vi "5.7.4-UDP-OCU_to_Forbrain-Client.vi"() -> ()   [LabVIEW 2010]
doc: "This VI implements a client for the Named Service UDP Server.vi.\nIt connects to a service by specifying the server address and the name of the service. After sending a 'Hello' string to the server, the client receives the string sent by the server, displays the string and closes the connection.\n\n<b>Note:</b> This VI is built to work with the Named Service UDP Server.vi in UDP.llb."
uses:
  6-OCU Neurons/AutoModeControls.ctl
  5.0-Global.vi
panel:
  out "AutoModeDatums":T1
  out "String":string
  out "error out":errorcluster
  in  "error in":errorcluster
  # "Instructions:\n1. Open Named Service UDP Server.vi located in the same library.\n2. Follow the instructions on it's front panel.\n\nNote: This VI is built to work with the Named Service UDP Server.vi in UDP.llb."
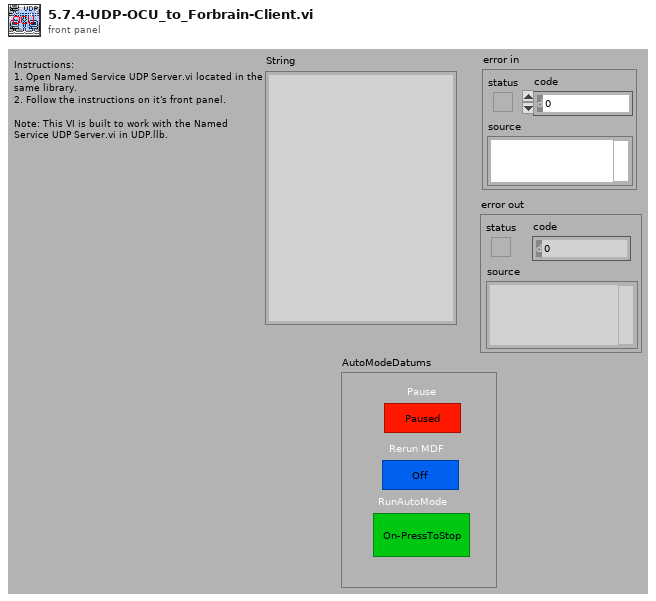
[diagram p1: front panel]
types:
  T1 = typedef "AutoModeControls.ctl" = cluster{"RunAutoMode":bool, "Rerun MDF":bool, "Pause":bool}
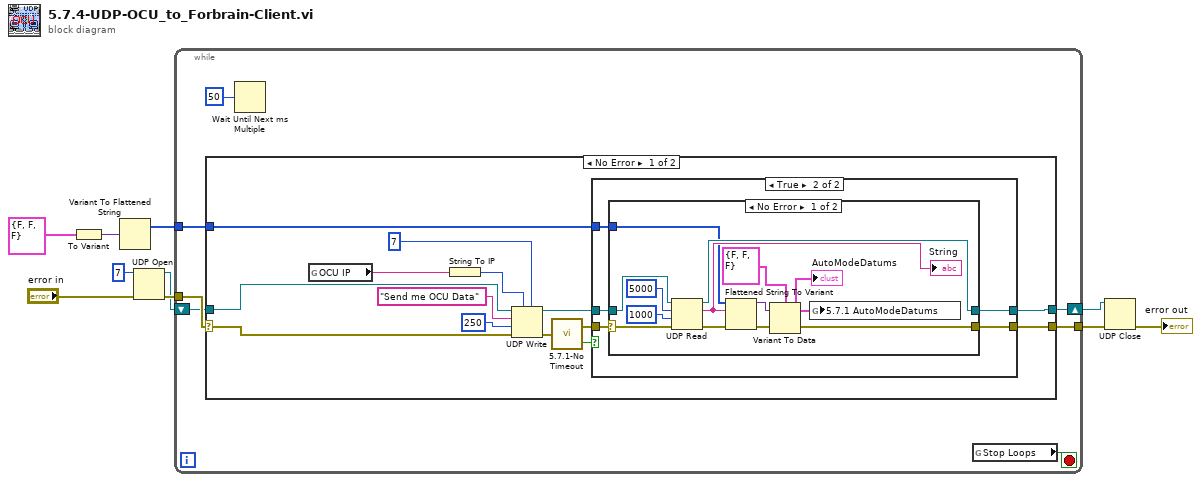
[diagram p0: block diagram]
diagram:
  n1 = To Variant(anything=T1 {"RunAutoMode"=FALSE, "Rerun MDF"=FALSE, "Pause"=FALSE} ("AutoModeDatums")) -> (Variant=w4:variant)
  n2 = Variant To Flattened String(Variant=w4) -> (1:w3:i16[])  [unwired: 1 out]
  n3 = UDP Open(8:"error in", 11:u16 7 ("port")) -> (port=w8:refnum<k16>, 0:w9:errorcluster)  [unwired: 3 in, 1 out]
  n4 = while {
    tunnel: [w17] -> w6
    tunnel: w9 -> [w16]
    shift-right: [w14] -> w7
    shift-left: w8 -> [w15]
    tunnel: w3 -> [w12]
    stop <- w11 stop-if-true
    n5 = case shown="No Error" w16 {
      selector: w16 -> [w31 w55]
      tunnel: [w26 w55] -> w17
      tunnel: w15 -> [w30 w54]
      tunnel: [w25 w54] -> w14
      tunnel: w12 -> [w20 _]
      frame No Error {
        n6 = global read "5.0-Global.vi" "OCU IP"() -> (w19:string)
        n7 = String To IP(1:w19) -> (0:w29:u32)
        n8 = UDP Write(address=w29, port or service name=u16 7, connection ID=w30, data in="Send me OCU Data", 8:w31, 9:250 ("timeout ms (25000)")) -> (error out=w24:errorcluster, 3:w27:refnum<k16>)
        n9 = call "5.7.1-No Timeout.vi"("error in (no error)"=w24) -> ("No Timeout"=w22:bool, "error out"=w23:errorcluster)
        n10 = case shown="True" w22 {
          tunnel: w23 -> [w33 w38]
          tunnel: w27 -> [w32 w37]
          tunnel: [w32 w36] -> w25
          tunnel: [w33 w35] -> w26
          tunnel: w20 -> [_ w34]
          frame False {
          }
          frame True {
            n11 = case shown="No Error" w38 {
              selector: w38 -> [w51 w52]
              tunnel: w37 -> [w50 w53]
              tunnel: [w48 w53] -> w36
              tunnel: [w41 w52] -> w35
              tunnel: w34 -> [w45 _]
              frame No Error {
                n12 = UDP Read(connection ID=w50, max size (548)=5000, timeout ms (25000)=1000, 8:w51) -> (data out=w46:string, error out=w42:errorcluster, 3:w48:refnum<k16>)  [unwired: 2 out]
                "String" <- w46
                n13 = Flattened String To Variant(4:w42, 6:w46, 7:w45) -> (0:w43:errorcluster, 3:w44:variant)
                n14 = Variant To Data(error in=w43, Variant=w44, type=T1 {"RunAutoMode"=FALSE, "Rerun MDF"=FALSE, "Pause"=FALSE} ("AutoModeDatums")) -> (error out=w41:errorcluster, data=w39:T1)
                "AutoModeDatums" <- w39
                n15 = global write "5.0-Global.vi" "5.7.1 AutoModeDatums"(w39) -> ()
              }
              frame Error {
              }
            }
          }
        }
      }
      frame Error {
      }
    }
    n16 = Wait Until Next ms Multiple(millisecond multiple=u32 50) -> ()  [unwired: 1 out]
    n17 = global read "5.0-Global.vi" "Stop Loops"() -> (w11:bool)
  }
  n18 = UDP Close(connection ID=w7, 8:w6) -> (error out=→"error out":errorcluster)  [unwired: 1 out]
